vi "Deadband Lifter.vi"(1 "Joystick Deadband Input":dbl) -> (0 "Joystick Deadband Output":dbl)   [LabVIEW 2015]
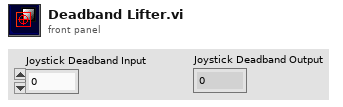
[diagram p1: front panel]
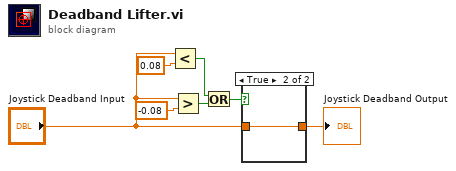
[diagram p0: block diagram]
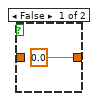
[diagram p2: hidden frame]
diagram:
  n1 = Less?(x="Joystick Deadband Input", y=0.08) -> (x < y?=w6:bool)
  n2 = Greater?(x="Joystick Deadband Input", y=-0.08) -> (0:w5:bool)
  n3 = Or(x=w6, y=w5) -> (x .or. y?=w4:bool)
  n4 = case shown="True" w4 {
    tunnel: [0.0 ("Joystick Arcband Input") w9] -> w7
    tunnel: "Joystick Deadband Input" -> [_ w9]
    frame False {
    }
    frame True {
    }
  }
  "Joystick Deadband Output" <- w7
